vi "Read Connection Status 2.vi"(11 "CCD in":refnum<class "CCD.lvclass">) -> (2 "Connection Status":bool, 3 "CCD out":refnum<class "CCD.lvclass">)   [LabVIEW 2016, in "Hardware.lvlib" / "CCD.lvlib" / "CCD.lvclass"]
uses:
  <userlib>/Common Components/Hardware/CCD/CCD/CCD.lvclass
  <userlib>/Common Components/Hardware/CCD/CCD/CCD.lvclass/CCD.ctl
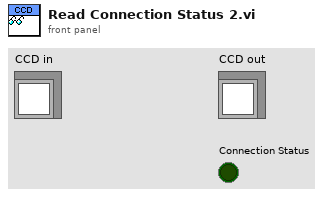
[diagram p1: front panel]
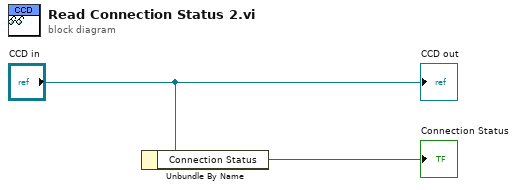
[diagram p0: block diagram]
diagram:
  n1 = Unbundle By Name("CCD in") -> ("Connection Status"=→"Connection Status":bool)
  "CCD out" <- "CCD in"
